vi "Relative Path.vi"() -> (1 "App\\LABVIEW":bool, 2 "Path":path)   [LabVIEW 2016]
panel:
  # "Relative Path.vi\n\nRitorna il path della directory dov'e' stato salvato, indipendentemente se chiamato da un eseguibile o no (VI di LabVIEW).\nUsando questo VI  per creare i path dei vari file utili ad un applicazione, non sarà poi necessario \nmodificare nulla creando l'eseguibile dell'applicazine.\n\nSe il VI viene salvato all'interno di directory che si trovano sotto una \"BIN\", ritornera' il path subito \"sopra\" la \"BIN\".\n - es \"C:\\app\\bin\\uno\\due\\tre\\Path.vi\"  ritornerà  \"c:\\app\"\nLo stesso vale se al posto di BIN si usano nomi che iniziano per BIN ( BINARY, BINS ...)\n\nCopyright (C) 2003 Alessandro Ricco - ale914@ilvg.it\n\n                                        Visita \"Italian LabVIEW user Group\" - www.ilvg.it\n\n\nThis library is free software; you can redistribute it and/or\nmodify it under the terms of the GNU Lesser General Public\nLicense as published by the Free Software Foundation; either\nversion 2.1 of the License, or (at your option) any later version.\nThis library is distributed in the hope that it will be useful,\nbut WITHOUT ANY WARRANTY; without even the implied warranty of\nMERCHANTABILITY or FITNESS FOR A PARTICULAR PURPOSE. See the GNU\nLesser General Public License for more details.\nYou should have received a copy of the GNU Lesser General Public\nLicense along with this library; if not, write to the Free Software\nFoundation, Inc., 59 Temple Place, Suite 330, Boston, MA 02111-1307 USA"
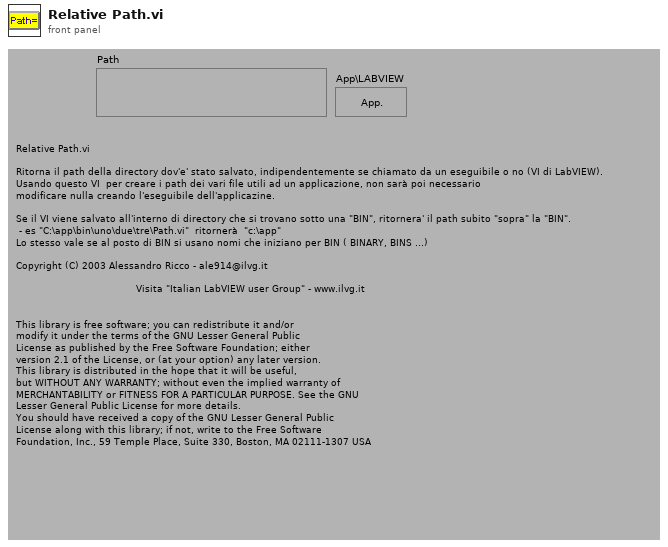
[diagram p1: front panel]
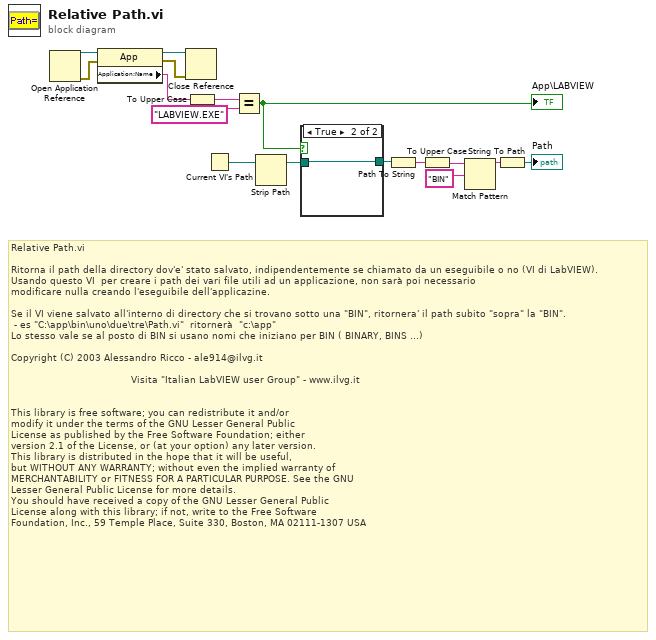
[diagram p0: block diagram]
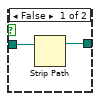
[diagram p2: hidden frame]
diagram:
  # "Relative Path.vi\n\nRitorna il path della directory dov'e' stato salvato, indipendentemente se chiamato da un eseguibile o no (VI di LabVIEW).\nUsando questo VI  per creare i path dei vari file utili ad un applicazione, non sarà poi necessario \nmodificare nulla creando l'eseguibile dell'applicazine.\n\nSe il VI viene salvato all'interno di directory che si trovano sotto una \"BIN\", ritornera' il path subito \"sopra\" la \"BIN\".\n - es \"C:\\app\\bin\\uno\\due\\tre\\Path.vi\"  ritornerà  \"c:\\app\"\nLo stesso vale se al posto di BIN si usano nomi che iniziano per BIN ( BINARY, BINS ...)\n\nCopyright (C) 2003 Alessandro Ricco - ale914@ilvg.it\n\n                                        Visita \"Italian LabVIEW user Group\" - www.ilvg.it\n\n\nThis library is free software; you can redistribute it and/or\nmodify it under the terms of the GNU Lesser General Public\nLicense as published by the Free Software Foundation; either\nversion 2.1 of the License, or (at your option) any later version.\nThis library is distributed in the hope that it will be useful,\nbut WITHOUT ANY WARRANTY; without even the implied warranty of\nMERCHANTABILITY or FITNESS FOR A PARTICULAR PURPOSE. See the GNU\nLesser General Public License for more details.\nYou should have received a copy of the GNU Lesser General Public\nLicense along with this library; if not, write to the Free Software\nFoundation, Inc., 59 Temple Place, Suite 330, Boston, MA 02111-1307 USA"
  n1 = Open Application Reference() -> (0:w3:errorcluster, 3:w8:refnum<vi>)  [unwired: 1 in, 3 out]
  n2 = property class="App"(reference=w8, error in=w3) -> (reference out=w1:refnum<vi>, error out=w2:errorcluster, "Application:Name"=w7:string)
  n3 = Close Reference(reference=w1, error in (no error)=w2) -> ()  [unwired: 1 out]
  n4 = To Upper Case(1:w7) -> (0:w4:string)
  n5 = Current VI's Path() -> (path=w16:path)
  n6 = Equal?(x=w4, y="LABVIEW.EXE") -> (x = y?=w5:bool)
  "App\\LABVIEW" <- w5
  n7 = Strip Path(path=w16) -> (stripped path=w10:path)  [unwired: 1 out]
  n8 = case shown="True" w5 {
    tunnel: w10 -> [w18 w19]
    tunnel: [w17 w19] -> w9
    frame False {
      n9 = Strip Path(path=w18) -> (stripped path=w17:path)  [unwired: 1 out]
    }
    frame True {
    }
  }
  n10 = Path To String(path=w9) -> (string=w15:string)
  n11 = To Upper Case(1:w15) -> (0:w14:string)
  n12 = Match Pattern(string=w14, regular expression="BIN") -> (before substring=w12:string)  [unwired: 4 out]
  n13 = String To Path(string=w12) -> (path=→"Path":path)
